vi "LIA_FPGA3a-PD Test-2.vi"() -> (1 "K Constant":fxp<+/-,32,16>, 2 "Nominal Freq":fxp<+/-,64,32>)   [LabVIEW 2012]
uses:
  <vilib>/rvi/DataTransferAndStorage/Container/Common/niFpgaContainerMetaDataKey.ctl
  <vilib>/rvi/DataTransferAndStorage/Container/Common/niFpgaContainerState.ctl
  <vilib>/rvi/DataTransferAndStorage/Container/Common/niFpgaDataTypeControl.ctl
  <vilib>/rvi/DataTransferAndStorage/Container/Common/niFpgaContainerImplementationControl.ctl
  <vilib>/rvi/DataTransferAndStorage/Container/Common/niFpgaContainerArbitrationOptionsControl.ctl
  <vilib>/rvi/DataTransferAndStorage/Container/Common/niFpgaTransferTypeControl.ctl
  <vilib>/rvi/DataTransferAndStorage/Container/Common/niFpgaContainerInitializationParameters.ctl
  <vilib>/rvi/Memory/Memory_Types/niFpgaMemoryInterfaceConfiguration.ctl
  <vilib>/rvi/FIFO/Fifo_Types/niFpgaFifoControlLogicControl.ctl
  <vilib>/Platform/TimedLoop/XDataNode/timing_clust.ctl
  <vilib>/Platform/TimedLoop/XDataNode/nitl_modes.ctl
  <vilib>/Platform/TimedLoop/XDataNode/wakeup.ctl
  <vilib>/rvi/FXPMathLib/FxpSinAndCos/subVIs/nifxpmath_SinAndCos_SimConfig.ctl
  <vilib>/rvi/FXPMathLib/basic elements/FxpIntAccumulator/subVIs/nifxpmath_IntAccumulator_SimConfig.ctl
  <vilib>/rvi/DataTransferAndStorage/Container/Common/niFpgaContainerGetUniqueNameForEmu.vi
  <vilib>/rvi/DataTransferAndStorage/Container/Common/niFpgaContainerSetEmuInfo.vi
  <vilib>/rvi/eio/common/nirviEmuReportErrorAndStop.vi
  <vilib>/rvi/FXPMathLib/FxpSinAndCos/simVIs/DllFxpSinAndCosTemp_sub.vi
  <vilib>/rvi/FXPMathLib/basic elements/FxpIntAccumulator/simVIs/DllFxpIntAccumulator_sub.vi
  <vilib>/rvi/eio/common/nirviEmuTemplateMethod_errors.vi
  <vilib>/rvi/Emulation/niFpgaSctlEmulationGetInTimedLoop.vi
  <vilib>/rvi/FIFO/Fifo_Resource/nirvififoEmulationSetSize.vi
  <vilib>/rvi/errors/niFpgaSetErrorForExecOnDevCompSimple.vi
  <vilib>/rvi/Emulation/niFpgaSctlEmulationFifoFullMgr.vi
  <vilib>/rvi/Emulation/niFpgaSctlEmulationResourceMgr.vi
  <vilib>/rvi/Emulation/niFpgaSctlEmulationRegisterWithScheduler.vi
  <vilib>/rvi/Emulation/niFpgaSctlEmulationScheduler.vi
  <vilib>/rvi/LocalResourceManager/LocalResourceManager.xnode
  <vilib>/Platform/TimedLoop/XDataNode/XDataNode.xnode
  <vilib>/rvi/FXPMathLib/FxpSinAndCos/XNode/nifxpmath_SinAndCos.xnode
  <vilib>/rvi/FXPMathLib/basic elements/FxpIntAccumulator/XNode/nifxpmath_IntAccumulator.xnode
  <vilib>/rvi/FXPMathLib/FxpInterpret/XNode/nifxpmath_Interpret.xnode
  <vilib>/eio/EIONode/EIONode.xnode
  <vilib>/rvi/DataTransferAndStorage/Container/XNode/niFpgaContainer.xnode
  <vilib>/rvi/FIFO/Fifo_Resource/nirvififoEmulationWrite.vi
  <vilib>/rvi/FIFO/Fifo_Resource/nirvififoEmulationRead.vi
  <vilib>/Platform/TimedLoop/XDataNode/XDNodeRunTimeDep.lvlib
panel:
  out "Test Input":fxp<+/-,64,32>
  out "Sine Output":fxp<+/-,64,32>
  in  "Voltage (V)":fxp<+,64,12>=3276.8125
  in  "Z":fxp<+/-,64,16>
  out "Summation":fxp<+/-,64,32>
  out "Test Output":i16
  in  "Test":i16
  out "Radians":fxp<+/-,14,5>
  out "Cos":fxp<+/-,14,2>
  out "Sin":fxp<+/-,14,2>
  in  "Period":u16=1000
  out "ticks":u16
  out "ref":i16 format="%.0x"
  out "sig":i16 format="%.0x"
  out "channelQ":i64
  out "channelI":i64
  out "f":fxp<+/-,32,0> format="%.32g"
  in  "start":bool
  in  "dec2":i16=1
  in  "K":fxp<+,16,0>=0.001007080078125
  in  "nominal freq":fxp<+,16,0>=0.010009765625
  in  "dec1":i16=1
  in  "stages":i8=1
  in  "stop":bool
  in  "decimation":i16=1024
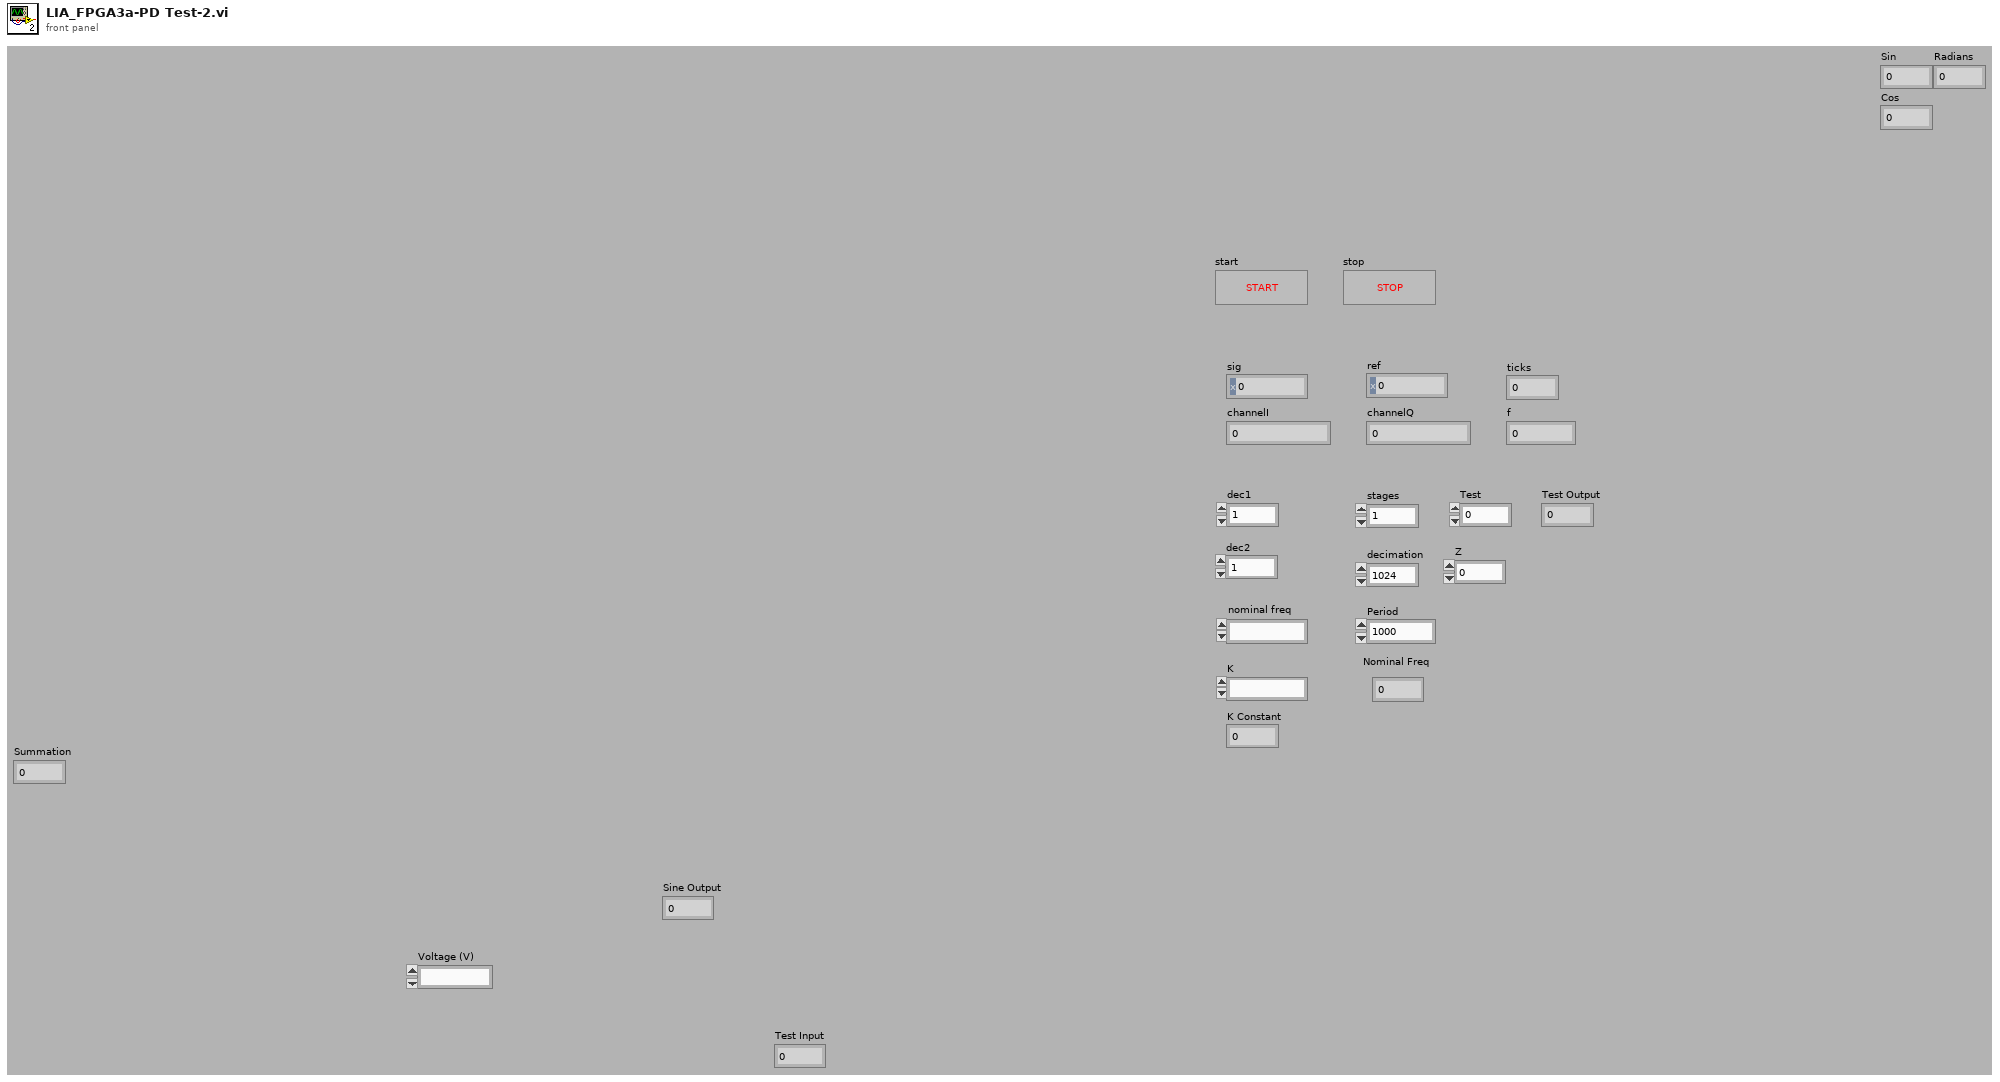
[diagram p1: front panel]
types:
  T1 = typedef "XDNodeRunTimeDep.lvlib/timing_clust.ctl" = cluster{"Expected End [f-1]":u64, "Actual End [f-1]":u64, "Finished Late? [f-1]":bool, "Expected End [i-1]":u64, "Actual End [i-1]":u64, "Finished Late? [i-1]":bool, "Expected Start [i]":u64, "Actual Start [i]":u64, "Expected Start [f]":u64, "Actual Start [f]":u64, "Source Name":string, "Structure Name":string, "Period":i64, "Deadline":i64, "Offset":i64, "Start":i64, "Priority":i32, "Timeout":i32, "Mode":T2, "Wakeup Reason":T3, "Error":errorcluster, "Source Type":string, "Secondary Source Type":string, "Global End Time":u64, "Global Start Time":u64, "Frame Duration":u64, "Iteration Duration":u64, "Assigned CPU":i32, "I/O Scan Engine Mode":u32}
  T2 = typedef "XDNodeRunTimeDep.lvlib/nitl_modes.ctl" = enum32{"No Change", "Process missed periods, maintain original phase", "Discard missed periods, maintain original phase", "Process missed periods, ignore original phase", "Discard missed periods, ignore original phase"}
  T3 = typedef "XDNodeRunTimeDep.lvlib/wakeup.ctl" = enum32{"Normal", "Aborted", "Asynchronous wakeup", "Timing source error", "Timed loop error", "Timeout"}
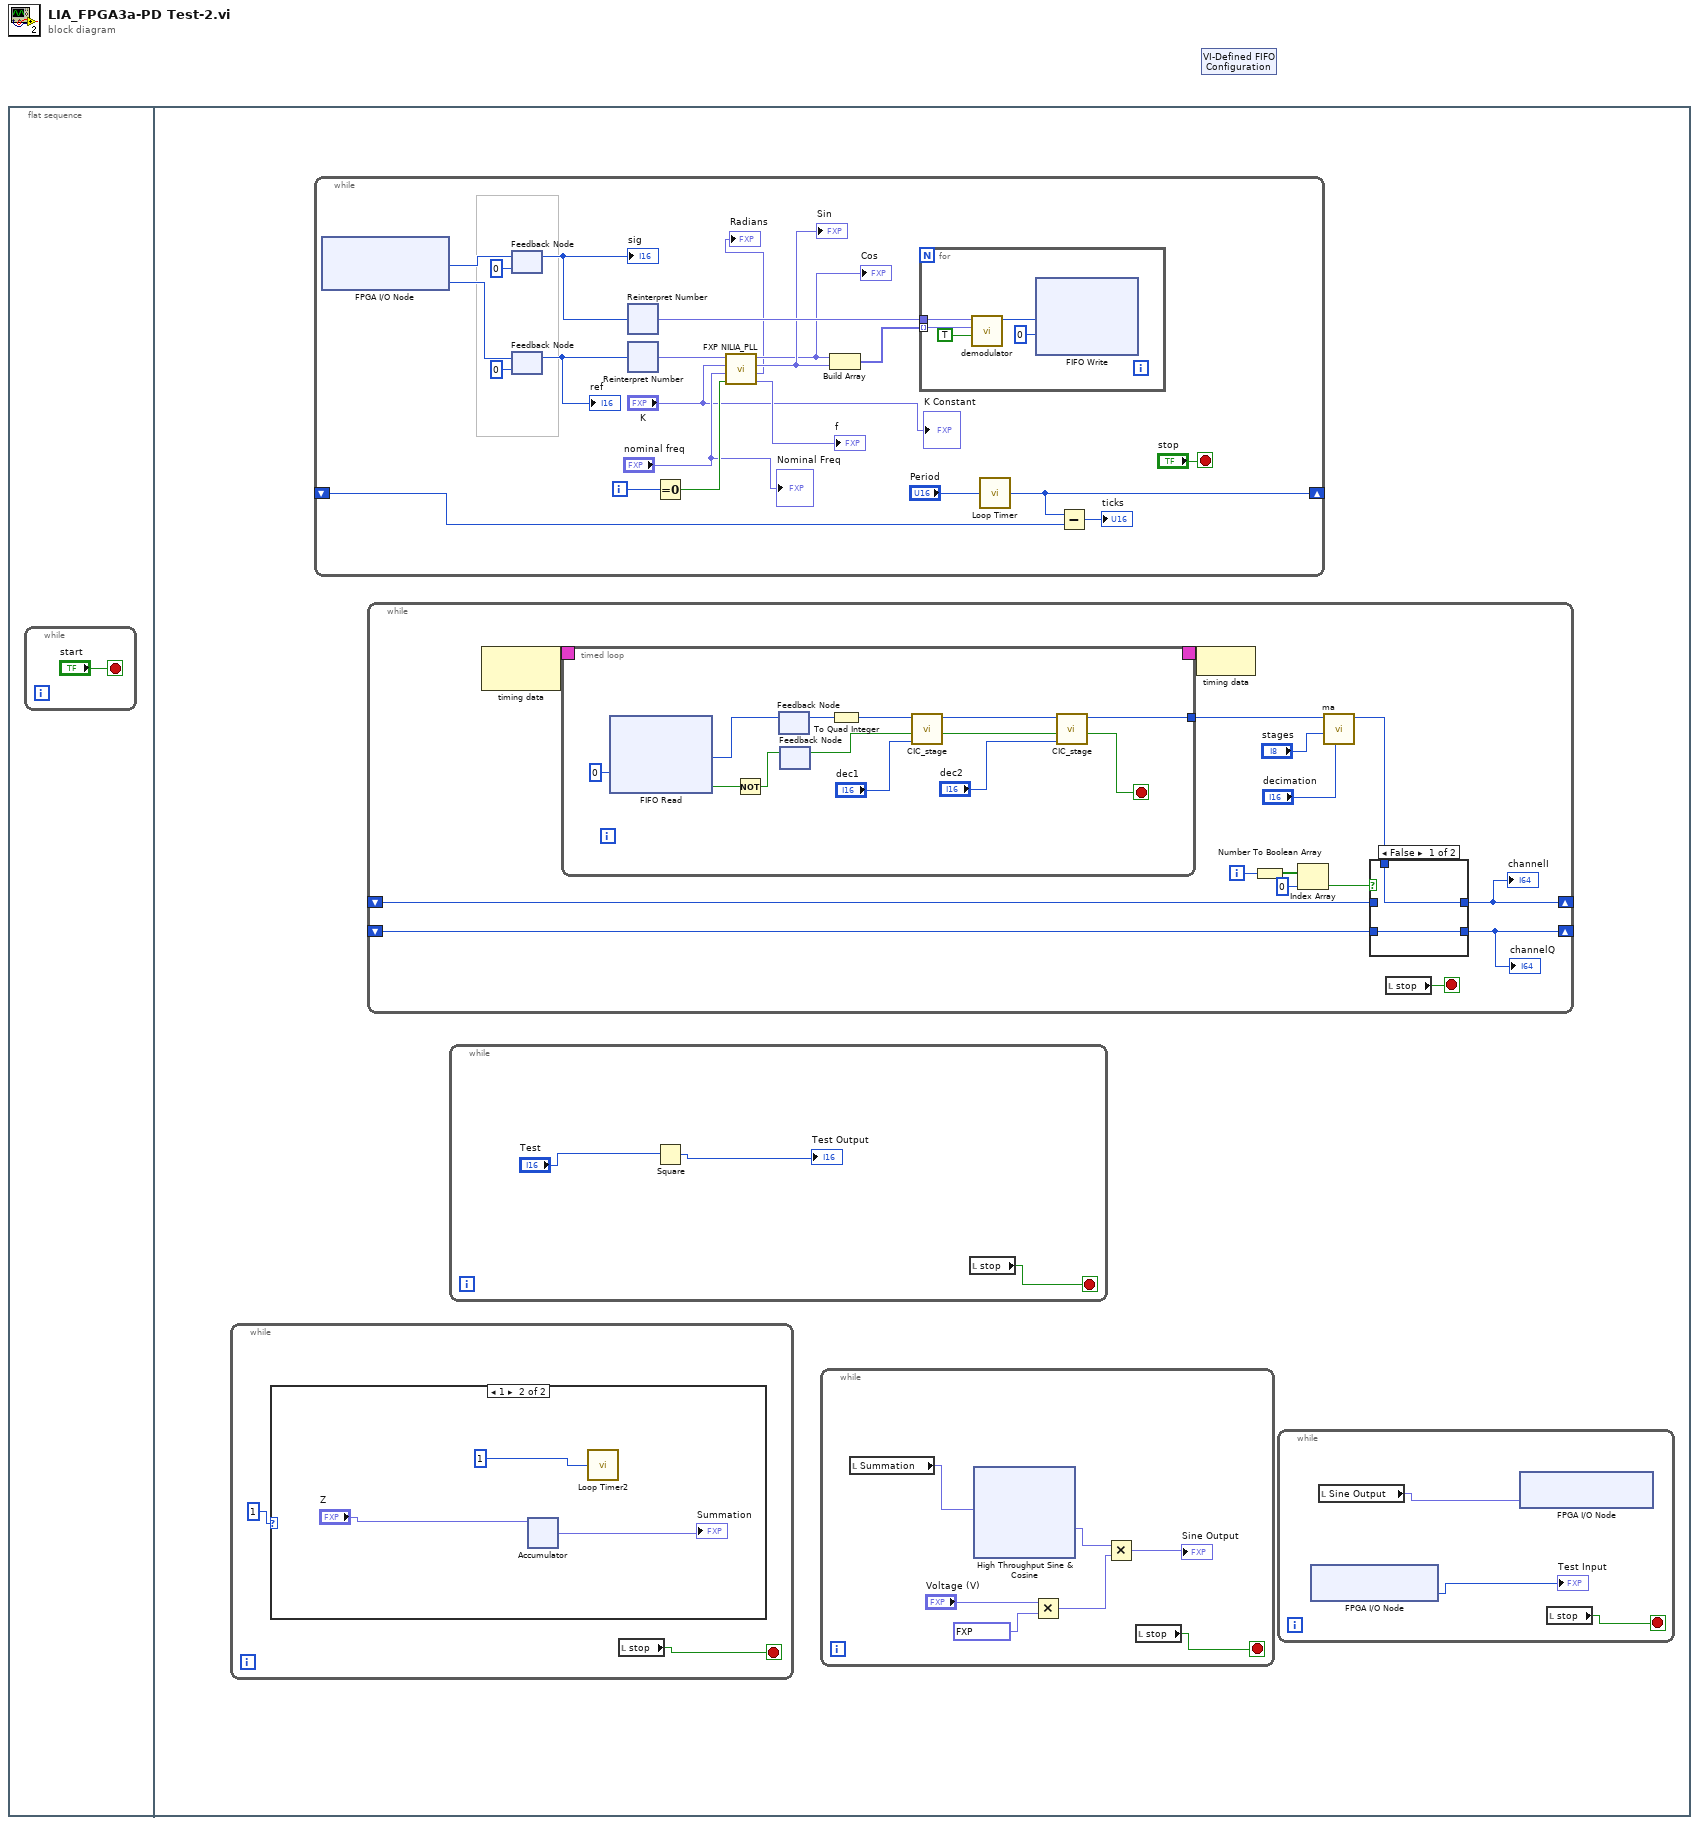
[diagram p0: block diagram]
diagram:
  n1 = flat-sequence {
    frame #0 {
      n2 = while {
        stop <- "start" stop-if-true
      }
    }
    frame #1 {
      n3 = while {
        stop <- w42 stop-if-true
        n4 = case shown="1" 1 {
          frame 0, Default {
          }
          frame 1 {
            n5 = xnode "Accumulator"("x"="Z") -> ("s"=→"Summation":fxp<+/-,64,16>)  [unwired: 4 in, 1 out]
            n6 = call "Loop Timer2"("Count(uSec)"=1) -> ()  [unwired: 1 out]
          }
        }
        n7 = local read "stop"() -> (w42:bool)
      }
      n8 = while {
        shift-right: [w95] -> _
        shift-left: _ -> [w94]
        i -> [w98]
        stop <- "stop" stop-if-true
        n9 = xnode "FPGA I/O Node"() -> ("Connector0/AI6"=w88:i16, "Connector0/AI7"=w85:i16)  [unwired: 2 in, 2 out]
        n10 = feedback #1(i16 0 ("y")) -> (w87:i16)
        "sig" <- w87
        n11 = feedback-in #1(w88) -> ()
        n12 = feedback #2(i16 0 ("z [I32.1]")) -> (w86:i16)
        "ref" <- w86
        n13 = feedback-in #2(w85) -> ()
        n14 = xnode "Reinterpret Number"("x"=w87) -> ("y"=w91:fxp<+/-,16,1>)
        n15 = xnode "Reinterpret Number"("x"=w86) -> ("y"=w84:fxp<+/-,16,1>)
        n16 = Equal To 0?(x=w98) -> (x = 0?=w82:bool)
        n17 = call "FXP NILIA_PLL.vi"("reset?"=w82, "norminal freq [U16.0]"="nominal freq", "alpha [U16.0]"="K", "x[I16.1]"=w84) -> ("f"=→"f":fxp<+/-,32,0>, "z [I32.1]"=→"Radians":fxp<+/-,32,1>, "sin(z)"=w79:fxp<+/-,16,2>, "cos(z)"=w78:fxp<+/-,16,2>)  [unwired: 4 in]
        "Sin" <- w79
        "Cos" <- w78
        n18 = Build Array(w78, w79) -> (w92:fxp<+/-,16,2>[])
        n19 = for {
          tunnel: w91 -> [w101]
          tunnel: w92 -> [w99] mode=indexing
          n20 = call "demodulator.vi"("New Data"=TRUE, "ref"=w99, "signal"=w101) -> ("x*y"=w102:i32)  [unwired: 8 out]
          n21 = xnode ("FIFO Write")("Element"=w102, "Timeout"=0) -> ()  [unwired: 1 in, 2 out]
        }
        n22 = call "Loop Timer"("Count(Ticks)"="Period") -> ("Tick Count(Ticks)"=w95:u16)
        n23 = Subtract(x=w95, y=w94) -> (x-y=→"ticks":u16)
        "Nominal Freq" <- "nominal freq"
        "K Constant" <- "K"
      }
      n24 = while {
        shift-right: [w105] -> _
        shift-left: _ -> [w107]
        shift-right: [w104] -> _
        shift-left: _ -> [w106]
        i -> [w112]
        stop <- w114 stop-if-true
        n25 = node-c288() -> (w118:T1)  [unwired: 1 out]
        n26 = timed-loop {
          timing: w118 -> [_]
          timing-out: [_] -> w117
          tunnel: [w126] -> w113
          stop <- w125 stop-if-true
          n27 = xnode ("FIFO Read")("Timeout"=0) -> ("Element"=w133:i32, "Timed Out?"=w132:bool)  [unwired: 1 in, 1 out]
          n28 = Not(x=w132) -> (.not. x?=w131:bool)
          n29 = feedback-in #3(w133) -> ()
          n30 = feedback #3() -> (w135:i32)  [unwired: 1 out]
          n31 = feedback-in #4(w131) -> ()
          n32 = feedback #4() -> (w129:bool)  [unwired: 1 out]
          n33 = To Quad Integer(1:w135) -> (0:w130:i64)
          n34 = call "CIC_stage.vi"("decimate factor"="dec1", "New Data"=w129, "input"=w130) -> ("Data Ready"=w127:bool, "output"=w128:i64)  [unwired: 7 out]
          n35 = call "CIC_stage.vi"("decimate factor"="dec2", "New Data"=w127, "input"=w128) -> ("Data Ready"=w125:bool, "output"=w126:i64)  [unwired: 7 out]
        }
        n36 = node-c288(w117) -> ()
        n37 = Number To Boolean Array(number=w112) -> (Boolean array=w111:bool[])
        n38 = Index Array "Index Array"(array=w111, index=0) -> (element=w109:bool)
        n39 = call "ma.vi"("decimate"="decimation", "stages"="stages", "input"=w113) -> ("output"=w108:i64)  [unwired: 8 out]
        n40 = case shown="False" w109 {
          tunnel: w108 -> [w120 w122]
          tunnel: [w120 w121] -> w105
          tunnel: [w119 w122] -> w104
          tunnel: w107 -> [_ w121]
          tunnel: w106 -> [w119 _]
          frame False {
          }
          frame True {
          }
        }
        "channelI" <- w105
        "channelQ" <- w104
        n41 = local read "stop"() -> (w114:bool)
      }
      n42 = while {
        stop <- w76 stop-if-true
        n43 = Square(x="Test") -> (x^2=→"Test Output":i16)
        n44 = local read "stop"() -> (w76:bool)
      }
      n45 = while {
        stop <- w5 stop-if-true
        n46 = local read "Summation"() -> (w11:fxp<+/-,64,32>)
        n47 = xnode "High Throughput Sine & Cosine"("x (pi)"=w11) -> ("sin(x)"=w10:fxp<+/-,16,2>)  [unwired: 1 out]
        n48 = Multiply(x="Voltage (V)", y=fxp<+,17,12> 3276.8125) -> (x*y=w6:fxp<+,64,24>)
        n49 = Multiply(x=w10, y=w6) -> (x*y=→"Sine Output":fxp<+/-,64,26>)
        n50 = local read "stop"() -> (w5:bool)
      }
      n51 = while {
        stop <- w2 stop-if-true
        n52 = xnode "FPGA I/O Node"() -> ("Connector0/AI5"=→"Test Input":i16)  [unwired: 1 in, 1 out]
        n53 = local read "Sine Output"() -> (w4:fxp<+/-,64,32>)
        n54 = xnode "FPGA I/O Node"("Connector0/AO2"=w4) -> ()  [unwired: 1 in, 1 out]
        n55 = local read "stop"() -> (w2:bool)
      }
    }
  }
  n56 = xnode "VI-Defined FIFO Configuration"() -> ()  [unwired: 1 out]
